vi "Save Section Index.vi"(8 "error in (no error)":errorcluster, 9 "Offset for index pointer":i32, 10 "File Section Offset":i32[](array[numeric])=[0], 11 "refnum":refnum<file>) -> (0 "error out":errorcluster, 3 "dup refnum":refnum<file>)   [LabVIEW 2009]
panel:
  out "offset":i32
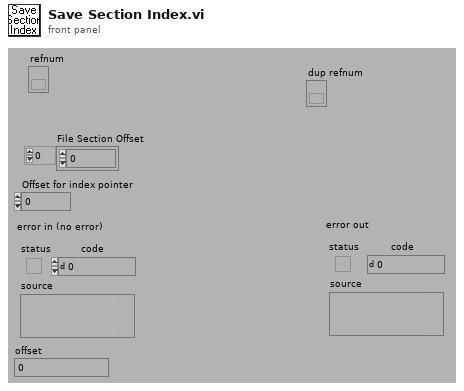
[diagram p1: front panel]
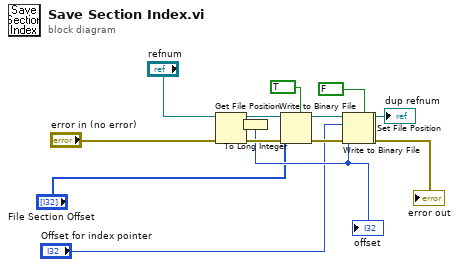
[diagram p0: block diagram]
diagram:
  n1 = Get File Position(4:"error in (no error)", 7:"refnum") -> (0:w16:errorcluster, 2:w1:i64, 3:w15:refnum<file>)
  n2 = To Long Integer(number=w1) -> (32bit integer=w13:i32)
  "offset" <- w13
  n3 = Write to Binary File(file (use dialog)=w15, data="File Section Offset", error in=w16, 5:TRUE ("header (F)")) -> (refnum out=w14:refnum<file>, error out=w12:errorcluster)  [unwired: 2 in, 1 out]
  n4 = Set File Position(offset (in bytes) (0)="Offset for index pointer", refnum=w14, error in=w12) -> (refnum out=w4:refnum<file>, error out=w3:errorcluster)  [unwired: 1 in]
  n5 = Write to Binary File(file (use dialog)=w4, data=w13, error in=w3, 5:FALSE ("prepend array or string size? (T)")) -> (refnum out=→"dup refnum":refnum<file>, error out=→"error out":errorcluster)  [unwired: 2 in, 1 out]
